vi "Quaternions to Euler.vi"(6 "Array":dbl[](array[numeric]), 9 "Array 2":dbl[](array[numeric]), 10 "Array 3":dbl[](array[numeric]), 11 "Array 4":dbl[](array[numeric])) -> (1 "Array 5":dbl[](array[numeric]), 2 "Array 6":dbl[](array[numeric]), 3 "Array 7":dbl[](array[numeric]))   [LabVIEW 2011]
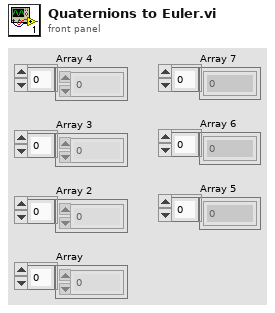
[diagram p1: front panel]
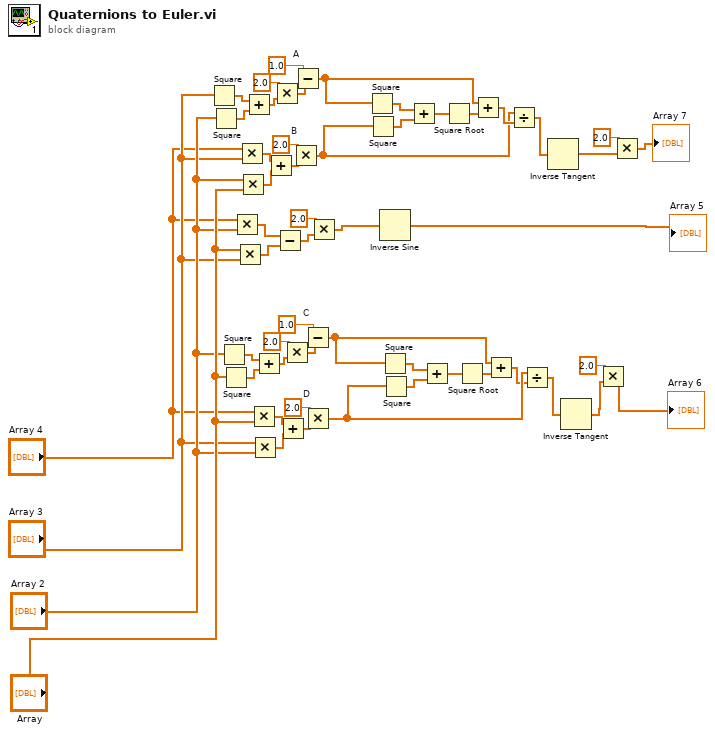
[diagram p0: block diagram]
diagram:
  n1 = Square(x="Array 3") -> (x^2=w11:dbl[])
  n2 = Square(x="Array 2") -> (x^2=w12:dbl[])
  n3 = Square(x="Array 2") -> (x^2=w17:dbl[])
  n4 = Square(x="Array") -> (x^2=w22:dbl[])
  n5 = Multiply(x="Array 4", y="Array 2") -> (x*y=w41:dbl[])
  n6 = Multiply(x="Array", y="Array 3") -> (x*y=w42:dbl[])
  n7 = Multiply(x="Array 4", y="Array 3") -> (x*y=w7:dbl[])
  n8 = Multiply(x="Array 2", y="Array") -> (x*y=w8:dbl[])
  n9 = Add(x=w11, y=w12) -> (x+y=w14:dbl[])
  n10 = Multiply(x="Array 4", y="Array") -> (x*y=w23:dbl[])
  n11 = Multiply(x="Array 3", y="Array 2") -> (x*y=w24:dbl[])
  n12 = Add(x=w17, y=w22) -> (x+y=w19:dbl[])
  n13 = Add(x=w7, y=w8) -> (x+y=w9:dbl[])
  n14 = Multiply(x=2.0, y=w14) -> (x*y=w16:dbl[])
  n15 = Subtract(x=w41, y=w42) -> (x-y=w44:dbl[])
  n16 = Add(x=w23, y=w24) -> (x+y=w25:dbl[])
  n17 = Multiply(x=2.0, y=w19) -> (x*y=w21:dbl[])
  n18 = Multiply "B"(x=2.0, y=w9) -> (x*y=w32:dbl[])
  n19 = Subtract "A"(x=1.0, y=w16) -> (x-y=w30:dbl[])
  n20 = Subtract "C"(x=1.0, y=w21) -> (x-y=w48:dbl[])
  n21 = Multiply "D"(x=2.0, y=w25) -> (x*y=w47:dbl[])
  n22 = Multiply(x=2.0, y=w44) -> (x*y=w45:dbl[])
  n23 = Square(x=w30) -> (x^2=w27:dbl[])
  n24 = Square(x=w32) -> (x^2=w28:dbl[])
  n25 = Inverse Sine(1:w45) -> (0:→"Array 5":dbl[])
  n26 = Square(x=w48) -> (x^2=w35:dbl[])
  n27 = Square(x=w47) -> (x^2=w36:dbl[])
  n28 = Add(x=w27, y=w28) -> (x+y=w29:dbl[])
  n29 = Add(x=w35, y=w36) -> (x+y=w37:dbl[])
  n30 = Square Root(x=w29) -> (sqrt(x)=w31:dbl[])
  n31 = Square Root(x=w37) -> (sqrt(x)=w38:dbl[])
  n32 = Add(x=w30, y=w31) -> (x+y=w33:dbl[])
  n33 = Add(x=w48, y=w38) -> (x+y=w39:dbl[])
  n34 = Divide(x=w32, y=w33) -> (x/y=w34:dbl[])
  n35 = Divide(x=w47, y=w39) -> (x/y=w40:dbl[])
  n36 = Inverse Tangent(1:w34) -> (0:w1:dbl[])
  n37 = Inverse Tangent(1:w40) -> (0:w5:dbl[])
  n38 = Multiply(x=2.0, y=w5) -> (x*y=→"Array 6":dbl[])
  n39 = Multiply(x=2.0, y=w1) -> (x*y=→"Array 7":dbl[])
